vi "iHR550 Read Values.vi"(1 "error in":errorcluster, 2 "JYMONOLib.IJYMonoReqd":refnum<k7>) -> (0 "iHR Current Values":T1={"iHR 550 Front Entrance"=0.0, "iHR550 Side Exit"=0.0, "iHR550 Wavelength"=897.9988, "iHR550 Exit Mirror"=2, "iHR550 Grating"="1", "Grating Index"=1} {"iHR550 Exit Mirror" items=["EntranceMirror", "ExitMirror", "Front", "Side"]})   [LabVIEW 2010]
uses:
  TypeDefs/iHR Current Values.ctl
panel:
  out "Current Description":string="1" caption="Description"
  out "Grating Index":i32=1
  out "Current Grating":dbl=1200.0
  out "error out":errorcluster
  out "Units 5":string="mm"
  out "Units 4":string="mm"
  out "Units 3":string="mm"
  out "Units 2":string="mm"
  out "Side Exit":dbl
  out "Front Exit":dbl
  out "Side Entrance":dbl
  out "Front Entrance":dbl
  out "Exit Mirror\nPosition":i32(ring)=2 items=["EntranceMirror", "ExitMirror", "Front", "Side"]
  out "Entrance Mirror\nPosition":i32(ring)=2 items=["EntranceMirror", "ExitMirror", "Front", "Side"]
  out "Units":string="nm"
  out "Current WL":dbl=897.9988
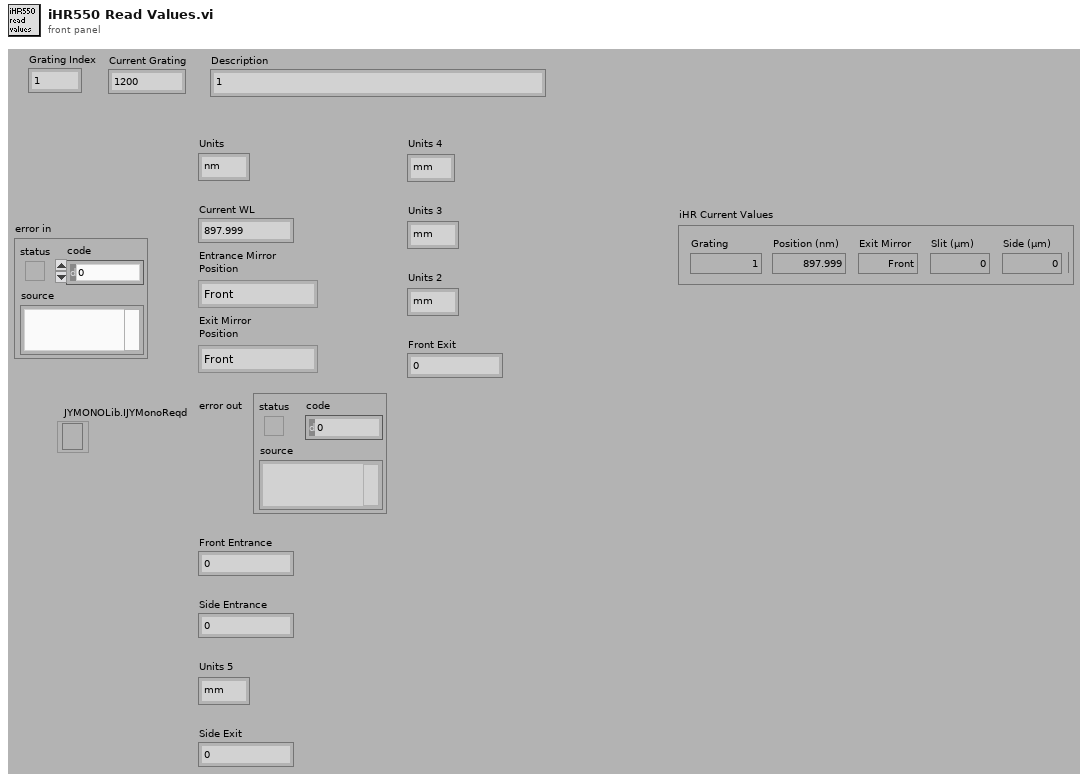
[diagram p1: front panel]
types:
  T1 = typedef "iHR Current Values.ctl" = cluster{"iHR 550 Front Entrance":dbl, "iHR550 Side Exit":dbl, "iHR550 Wavelength":dbl, "iHR550 Exit Mirror":i32, "iHR550 Grating":string, "Grating Index":i32}
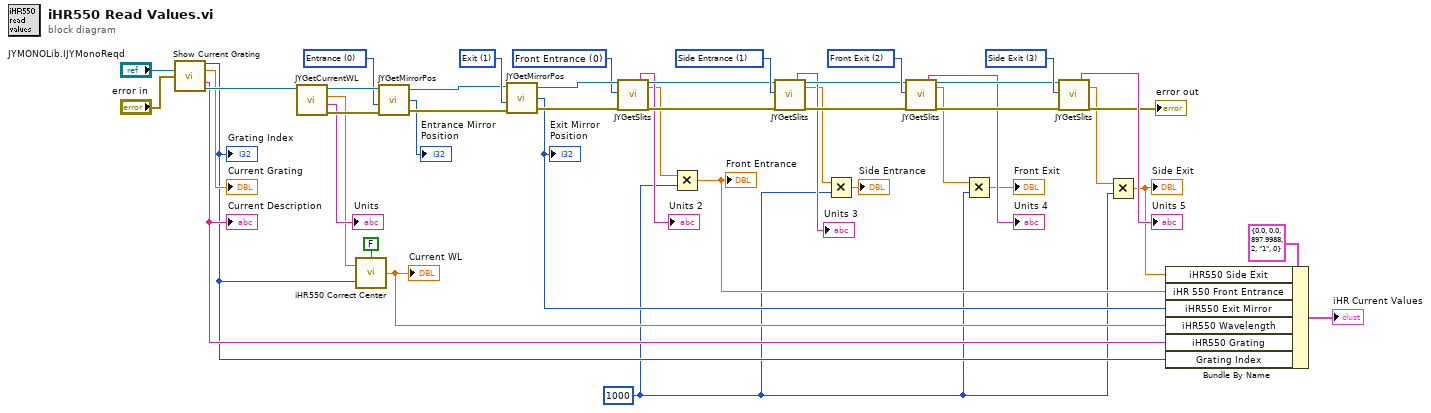
[diagram p0: block diagram]
diagram:
  w5 = i16 1000 ("y")
  w41 = u16 3 items=["Front Entrance", "Side Entrance", "Front Exit", "Side Exit", "First Intermediate", "Second Intermediate"] ("Slit")
  w42 = u16 2 items=["Front Entrance", "Side Entrance", "Front Exit", "Side Exit", "First Intermediate", "Second Intermediate"] ("Slit")
  w43 = u16 1 items=["Front Entrance", "Side Entrance", "Front Exit", "Side Exit", "First Intermediate", "Second Intermediate"] ("Slit")
  w44 = u16 0 items=["Front Entrance", "Side Entrance", "Front Exit", "Side Exit", "First Intermediate", "Second Intermediate"] ("Slit")
  w26 = u16 1 items=["Entrance", "Exit"] ("Mirror Number")
  w27 = u16 0 items=["Entrance", "Exit"] ("Mirror Number")
  n1 = call "Show Current Grating.vi"("Refnum in"="JYMONOLib.IJYMonoReqd", "error in (no error)"="error in") -> ("Grating Index"=w10:i32, "Current Grating"=→"Current Grating":dbl, "Current Description"=w15:string, "JYMONOLib.IJYMonoReqd"=w19:refnum<k7>)  [unwired: 5 in, 5 out]
  "Grating Index" <- w10
  "Current Description" <- w15
  n2 = call "JYGetCurrentWL.vi"("JYMONOLib.IJYMonoReqd"=w19) -> ("error out"=w29:errorcluster, "Units"=→"Units":string, "Current WL"=w11:dbl, "JYMONOLib.IJYMonoReqd 2"=w28:refnum<k7>)  [unwired: 7 in]
  n3 = call "iHR550 Correct Center.vi"("Set?"=FALSE, "Grating Index"=w10, "Position In (nm)"=w11) -> ("Position Out (nm)"=w12:dbl)
  "Current WL" <- w12
  n4 = call "JYGetMirrorPos.vi"("error in (no error)"=w29, "Mirror"=w27, "Refnum In"=w28) -> ("error out"=w24:errorcluster, "Current Mirror Position"=→"Entrance Mirror\nPosition":i32, "Refnum Out"=w25:refnum<k7>)  [unwired: 1 in]
  n5 = call "JYGetMirrorPos.vi"("error in (no error)"=w24, "Mirror"=w26, "Refnum In"=w25) -> ("error out"=w45:errorcluster, "Current Mirror Position"=w16:i32, "Refnum Out"=w46:refnum<k7>)  [unwired: 1 in]
  "Exit Mirror\nPosition" <- w16
  n6 = call "JYGetSlits.vi"("MonoRefNum IN"=w46, "Slit"=w44, "error in (no error)"=w45) -> ("Units"=→"Units 2":string, "MonoRefNum Out"=w40:refnum<k7>, "Slit Width"=w9:dbl, "error out"=w37:errorcluster)  [unwired: 13 in]
  n7 = Multiply(x=w9, y=w5) -> (x*y=w6:dbl)
  "Front Entrance" <- w6
  n8 = call "JYGetSlits.vi"("MonoRefNum IN"=w40, "Slit"=w43, "error in (no error)"=w37) -> ("Units"=→"Units 3":string, "MonoRefNum Out"=w39:refnum<k7>, "Slit Width"=w8:dbl, "error out"=w36:errorcluster)  [unwired: 13 in]
  n9 = Multiply(x=w8, y=w5) -> (x*y=→"Side Entrance":dbl)
  n10 = call "JYGetSlits.vi"("MonoRefNum IN"=w39, "Slit"=w42, "error in (no error)"=w36) -> ("Units"=→"Units 4":string, "MonoRefNum Out"=w38:refnum<k7>, "Slit Width"=w1:dbl, "error out"=w35:errorcluster)  [unwired: 13 in]
  n11 = Multiply(x=w1, y=w5) -> (x*y=→"Front Exit":dbl)
  n12 = call "JYGetSlits.vi"("MonoRefNum IN"=w38, "Slit"=w41, "error in (no error)"=w35) -> ("Units"=→"Units 5":string, "Slit Width"=w2:dbl, "error out"=→"error out":errorcluster)  [unwired: 13 in, 1 out]
  n13 = Multiply(x=w2, y=w5) -> (x*y=w3:dbl)
  "Side Exit" <- w3
  n14 = Bundle By Name(cluster=T1 {"iHR 550 Front Entrance"=0.0, "iHR550 Side Exit"=0.0, "iHR550 Wavelength"=897.9988, "iHR550 Exit Mirror"=2, "iHR550 Grating"="1", "Grating Index"=0} ("iHR Current Values"), "iHR550 Side Exit"=w3, "iHR 550 Front Entrance"=w6, "iHR550 Exit Mirror"=w16, "iHR550 Wavelength"=w12, "iHR550 Grating"=w15, "Grating Index"=w10) -> (→"iHR Current Values":T1)
